vi "ignore some errors.vi"(5 "max errors":i32=1, 6 "reset":bool, 7 "error code":i32, 8 "error in":errorcluster) -> (0 "error out":errorcluster, 3 "errors":i32)   [LabVIEW 2012]
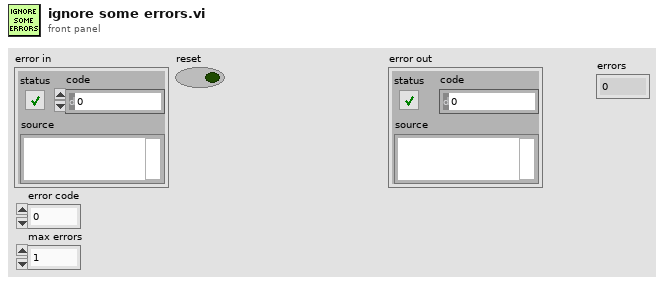
[diagram p1: front panel]
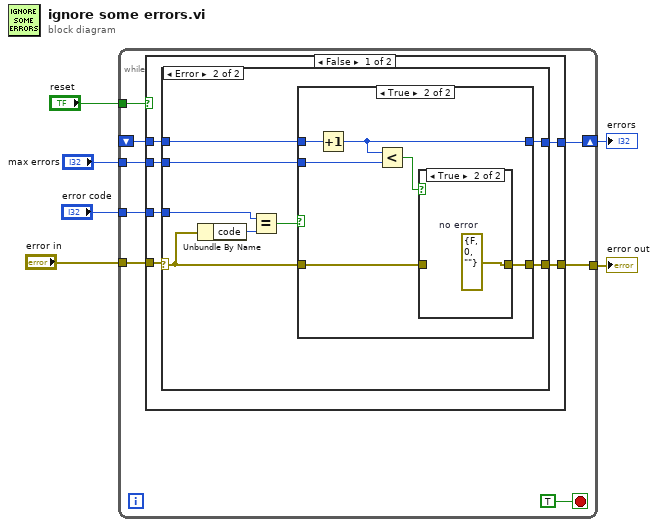
[diagram p0: block diagram]
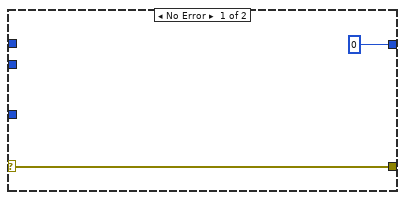
[diagram p2: hidden frame]
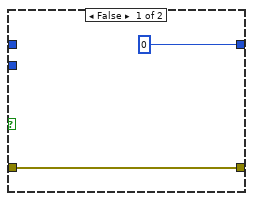
[diagram p3: hidden frame]
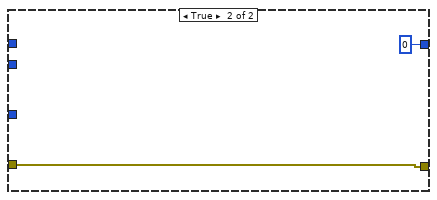
[diagram p5: hidden frame]
diagram:
  n1 = while {
    shift-right: [w13] -> w1
    shift-left: _ -> [w11]
    tunnel: "error in" -> [w14]
    tunnel: "error code" -> [w12]
    tunnel: [w10] -> w4
    tunnel: "max errors" -> [w9]
    tunnel: "reset" -> [w7]
    stop <- TRUE stop-if-true
    n2 = case shown="False" w7 {
      tunnel: w14 -> [w20 w41]
      tunnel: [w19 0] -> w13
      tunnel: w12 -> [w18 _]
      tunnel: w11 -> [w17 _]
      tunnel: [w16 w41] -> w10
      tunnel: w9 -> [w15 _]
      frame False {
        n3 = case shown="Error" w20 {
          selector: w20 -> [w21 w25]
          tunnel: [0 w26] -> w19
          tunnel: w18 -> [_ w29]
          tunnel: w17 -> [_ w27]
          tunnel: [w21 w24] -> w16
          tunnel: w15 -> [_ w23]
          frame No Error {
          }
          frame Error {
            n4 = Unbundle By Name(w25) -> ("code"=w30:i32)
            n5 = Equal?(x=w29, y=w30) -> (x = y?=w28:bool)
            n6 = case shown="True" w28 {
              tunnel: w27 -> [_ w38]
              tunnel: [0 w36] -> w26
              tunnel: w25 -> [w31 w33]
              tunnel: [w31 w37] -> w24
              tunnel: w23 -> [_ w35]
              frame False {
              }
              frame True {
                n7 = Increment(x=w38) -> (x+1=w36:i32)
                n8 = Less?(x=w36, y=w35) -> (x < y?=w34:bool)
                n9 = case shown="True" w34 {
                  tunnel: [w39 w40] -> w37
                  tunnel: w33 -> [w39 _]
                  frame False {
                  }
                  frame True {
                    w40 = errorcluster {"status"=FALSE, "code"=0, "source"=""}  # no error
                  }
                }
              }
            }
          }
        }
      }
      frame True {
      }
    }
  }
  "error out" <- w4
  "errors" <- w1
